vi "Create IO Control.vi"(8 "error in (no error)":errorcluster, 10 "IO Control":T2 {"Signals"."Response"."Byte Order" items=["Little Endian", "Big Endian"]; "Signals"."Response"."Data Type" items=["Signed", "Unsigned", "IEEE Float"]; "Signals"."Cmd"."Byte Order" items=["Little Endian", "Big Endian"]; "Signals"."Cmd"."Data Type" items=["Signed", "Unsigned", "IEEE Float"]}, 11 "Section Ptr":T1 format="%.0x") -> (0 "error out":errorcluster, 3 "Parent Ref out":T1 format="%.0x")   [LabVIEW 2015, in "Diagnostics Addon Shared.lvlib"]
uses:
  Diagnostics Addon Shared.lvlib
  IO Control Parameters.ctl
  Input and Output Signal Parameters.ctl
  DIDPID Signal Parameters.ctl
  <vilib>/NI Veristand/Custom Device API/Custom Device Item Ref.ctl
  FG Action.ctl
  <vilib>/NI Veristand/Custom Device API/NI VeriStand - Get Item Property.vi
  <vilib>/NI Veristand/Custom Device API/Get Item Property (U32).vi
  <vilib>/NI Veristand/Custom Device API/NI VeriStand - Set Item Property.vi
  <vilib>/NI Veristand/Custom Device API/Set Item Property (U32).vi
  GUID Lookup.vi
  <vilib>/NI Veristand/Custom Device API/Custom Device API.lvlib
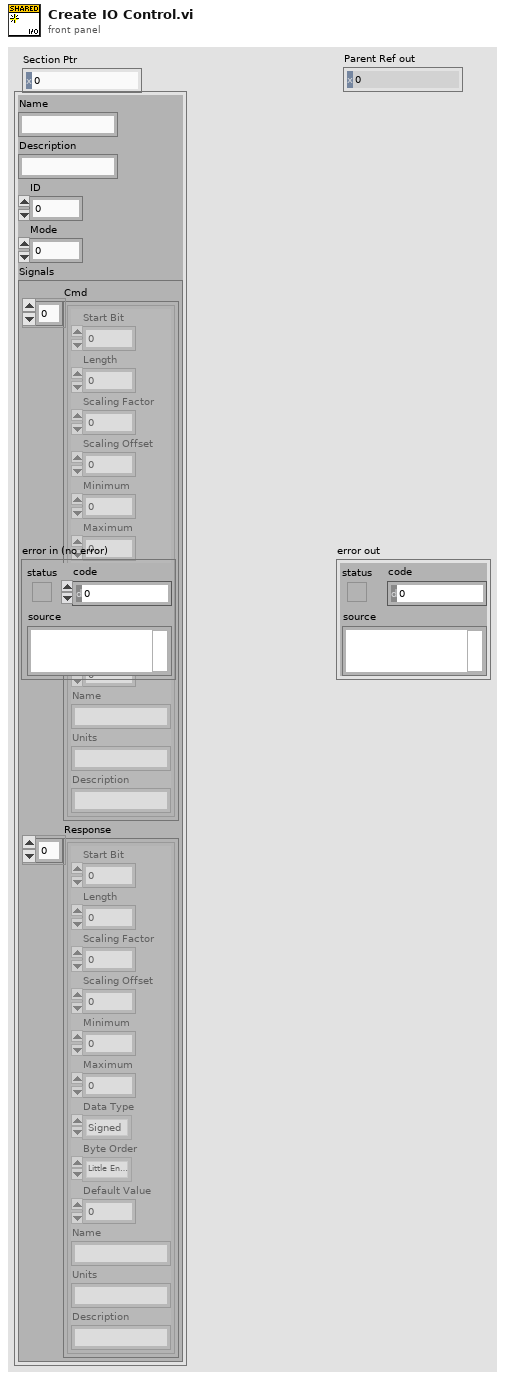
[diagram p1: front panel]
types:
  T1 = typedef "Custom Device API.lvlib/Custom Device Item Ref.ctl" = u64
  T2 = typedef "Diagnostics Addon Shared.lvlib/IO Control Parameters.ctl" = cluster{"Name":string, "Description":string, "ID":u16, "Mode":u8, "Signals":T3}
  T3 = typedef "Diagnostics Addon Shared.lvlib/Input and Output Signal Parameters.ctl" = cluster{"Cmd":T4[], "Response":T4[]}
  T4 = typedef "Diagnostics Addon Shared.lvlib/DIDPID Signal Parameters.ctl" = cluster{"Start Bit":u8, "Length":u8, "Scaling Factor":dbl, "Scaling Offset":dbl, "Minimum":dbl, "Maximum":dbl, "Data Type":u32, "Byte Order":u32, "Default Value":dbl, "Name":string, "Units":string, "Description":string}
  T5 = typedef "Diagnostics Addon Shared.lvlib/FG Action.ctl" = enum16{"Get", "Set"}
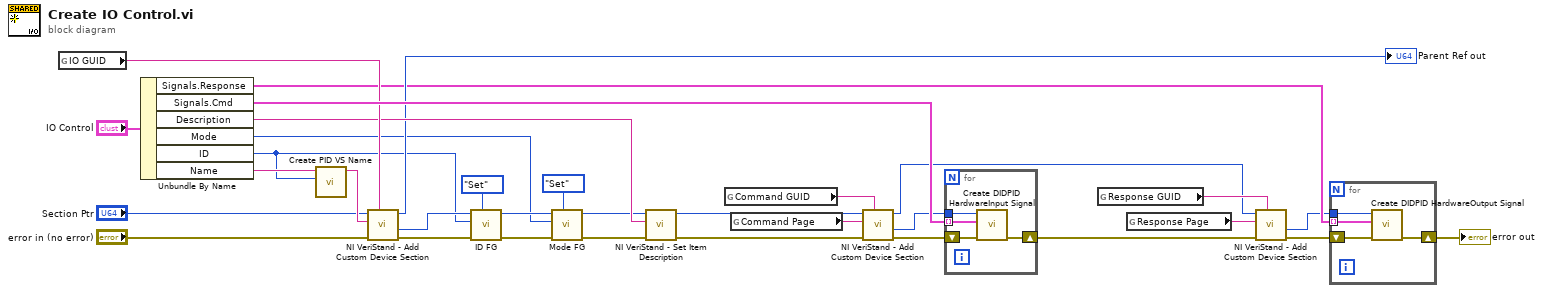
[diagram p0: block diagram]
diagram:
  n1 = global read "GUID Lookup.vi" "IO GUID"() -> (w30:string)
  n2 = Unbundle By Name("IO Control") -> ("Signals.Response"=w24:T4[], "Signals.Cmd"=w32:T4[], "Description"=w27:string, "Mode"=w2:u8, "ID"=w8:u16, "Name"=w11:string)
  n3 = call "Create PID VS Name.vi"("PID Number"=w8, "PID Name"=w11) -> ("VS Name"=w33:string)  [unwired: 9 in]
  n4 = call <vilib>:"NI VeriStand - Add Custom Device Section.vi"("GUID (Default Section)"=w30, "error in (no error)"="error in (no error)", "Section Name"=w33, "Parent Ref in"="Section Ptr") -> ("error out"=w10:errorcluster, "Section Ptr"=w9:T1, "Parent Ref out"=→"Parent Ref out":T1)  [unwired: 4 in, 1 out]
  n5 = call "ID FG.vi"("Action"=FG_Action."Set", "error in (no error)"=w10, "ID"=w8, "Device Item Ref in"=w9) -> ("error out"=w7:errorcluster, "Device Item Ref out"=w4:T1)  [unwired: 5 in, 1 out]
  n6 = call "Mode FG.vi"("Action"=FG_Action."Set", "error in (no error)"=w7, "Mode"=w2, "Device Item Ref in"=w4) -> ("error out"=w6:errorcluster, "Device Item Ref out"=w3:T1)  [unwired: 5 in, 1 out]
  n7 = call <vilib>:"NI VeriStand - Set Item Description.vi"("error in (no error)"=w6, "Description"=w27, "Item Ref in"=w3) -> ("error out"=w18:errorcluster, "Item Ref out"=w17:T1)  [unwired: 6 in, 1 out]
  n8 = global read "GUID Lookup.vi" "Command GUID"() -> (w22:string)
  n9 = global read "GUID Lookup.vi" "Command Page"() -> (w23:string)
  n10 = call <vilib>:"NI VeriStand - Add Custom Device Section.vi"("GUID (Default Section)"=w22, "error in (no error)"=w18, "Section Name"=w23, "Parent Ref in"=w17) -> ("error out"=w15:errorcluster, "Section Ptr"=w14:T1, "Parent Ref out"=w19:T1)  [unwired: 4 in, 1 out]
  n11 = for {
    shift-right: [w36] -> w16
    shift-left: w15 -> [w37]
    tunnel: w32 -> [w34] mode=indexing
    tunnel: w14 -> [w35]
    n12 = call "Create DIDPID HardwareInput Signal.vi"("error in (no error)"=w37, "Signal Parameters"=w34, "Section Ptr"=w35) -> ("error out"=w36:errorcluster)  [unwired: 7 in, 1 out]
  }
  n13 = global read "GUID Lookup.vi" "Response GUID"() -> (w21:string)
  n14 = global read "GUID Lookup.vi" "Response Page"() -> (w20:string)
  n15 = call <vilib>:"NI VeriStand - Add Custom Device Section.vi"("GUID (Default Section)"=w21, "error in (no error)"=w16, "Section Name"=w20, "Parent Ref in"=w19) -> ("error out"=w13:errorcluster, "Section Ptr"=w12:T1)  [unwired: 4 in, 2 out]
  n16 = for {
    shift-right: [w38] -> w25
    shift-left: w13 -> [w40]
    tunnel: w24 -> [w39] mode=indexing
    tunnel: w12 -> [w41]
    n17 = call "Create DIDPID HardwareOutput Signal.vi"("error in (no error)"=w40, "Signal Parameters"=w39, "Section Ptr"=w41) -> ("error out"=w38:errorcluster)  [unwired: 7 in, 1 out]
  }
  "error out" <- w25
